vi "NovaTech409A_Close.vi"(2 "error in (no error)":errorcluster, 3 "VISA resource name":refnum<visa-resource-name>="COM1") -> (0 "error out":errorcluster)   [LabVIEW 2013, in "Novatech 409A.lvlib"]
uses:
  Novatech 409A.lvlib
panel:
  out "read buffer 1":string="OK\r\n"
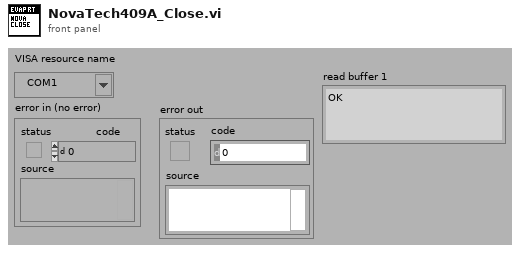
[diagram p1: front panel]
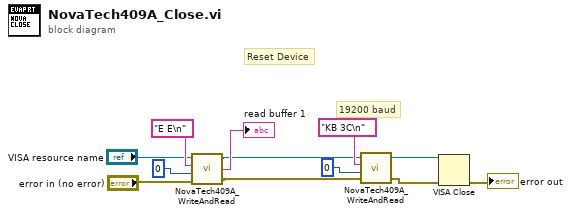
[diagram p0: block diagram]
diagram:
  # "19200 baud"
  # "Reset Device"
  n1 = call "NovaTech409A_WriteAndRead.vi"("error in (no error)"="error in (no error)", "Number of Bytes"=0, "write buffer"="E E\n", "VISA resource name"="VISA resource name") -> ("error out"=w2:errorcluster, "read buffer"=→"read buffer 1":string, "VISA resource name out"=w1:refnum<visa-resource-name>)
  n2 = call "NovaTech409A_WriteAndRead.vi"("error in (no error)"=w2, "Number of Bytes"=0, "write buffer"="KB 3C\n", "VISA resource name"=w1) -> ("error out"=w3:errorcluster, "VISA resource name out"=w4:refnum<visa-resource-name>)  [unwired: 1 out]
  n3 = VISA Close(VISA resource name=w4, error in (no error)=w3) -> (error out=→"error out":errorcluster)
